vi "init.vi"(8 "error in (no error)":errorcluster, 10 "Variant":variant, 11 "Arduino Uno in":refnum<class "Arduino Uno.lvclass">) -> (0 "error out":errorcluster, 3 "Arduino Uno out":refnum<class "Arduino Uno.lvclass">)   [LabVIEW 2025, in "USB IO.lvlib" / "Arduino Uno.lvclass"]
uses:
  Arduino Uno.lvclass
  Arduino Uno.lvclass/Arduino Uno.ctl
  <vilib>/MakerHub/LINX/Public/Utilities/Open Serial.vi
  <vilib>/MakerHub/LINX/LMH-LINX.lvlib
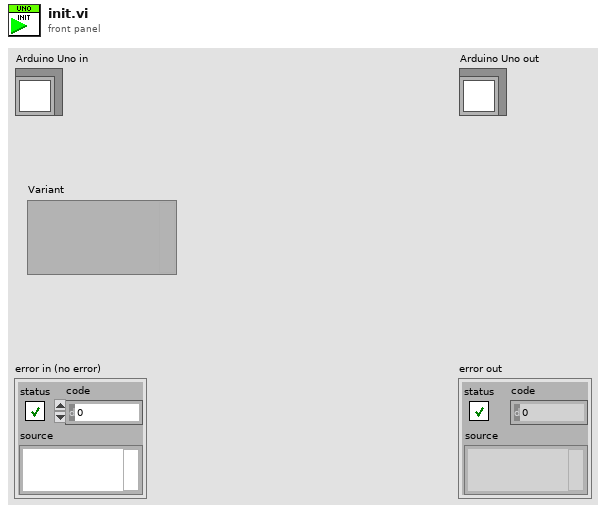
[diagram p1: front panel]
types:
  T1 = typedef "LMH-LINX.lvlib/LINX Ref.ctl" = cluster{"IO":T2, "Interface":T3, "LINX Device Config":T4}
  T2 = typedef "LMH-LINX.lvlib/Platform.ctl" = enum16{"Remote", "Local"}
  T3 = typedef "LMH-LINX.lvlib/Interface.ctl" = enum16{"Serial", "TCP"}
  T4 = typedef "LMH-LINX.lvlib/Device.lvlib/LINX Device Config.ctl" = cluster{"Interface":T3, "COM Port":refnum<visa-resource-name>, "TCP Configuration":T5, "Device Family":u8, "Device ID":u8, "Device Name":string, "TCP Ref":refnum<k5>, "Channels":T6}
  T5 = typedef "LMH-LINX.lvlib/Device.lvlib/TCP Config.ctl" = cluster{"IP Address":string, "Port":u16}
  T6 = typedef "LMH-LINX.lvlib/Channels.ctl" = cluster{"DI":u8[], "DO":u8[], "AI":u8[], "AO":u8[], "PWM":u8[], "QE":u8[], "UART":u8[], "I2C 2":u8[], "SPI":u8[], "CAN":u8[], "Servo":u8[], "AI Ref (V)":dbl, "AI Resolution (Bits)":u8, "AO Ref (V)":dbl, "AO Resolution (Bits)":u8}
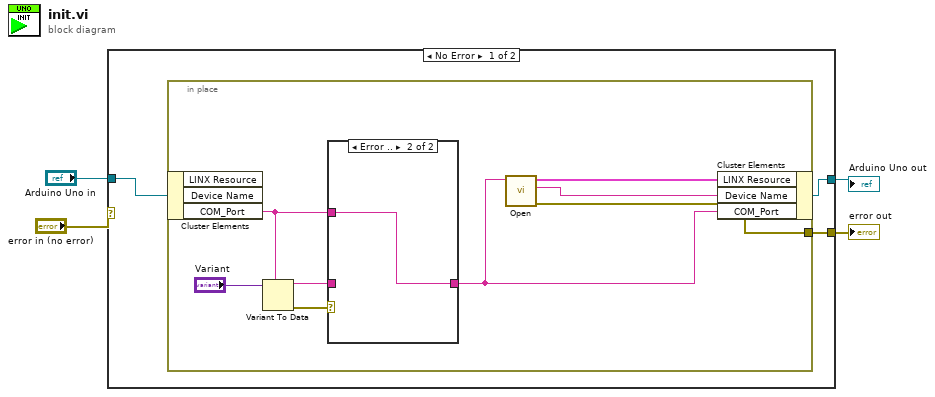
[diagram p0: block diagram]
diagram:
  n1 = case shown="No Error" "error in (no error)" {
    selector: "error in (no error)" -> [_ w18]
    tunnel: "Arduino Uno in" -> [w7 w19]
    tunnel: [w6 w18] -> w2
    tunnel: [w5 w19] -> w1
    frame No Error {
      n2 = in-place {
        in-place-border: [w14] -> w6
        n3 = in-place-cluster #1(w7) -> ("COM_Port"=w9:string)  [unwired: 2 out]
        n4 = Variant To Data(type=w9, Variant="Variant") -> (data=w10:string, error out=w11:errorcluster)  [unwired: 1 in]
        n5 = case shown="Error .." w11 {
          tunnel: w10 -> [w16 _]
          tunnel: [w16 w17] -> w8
          tunnel: w9 -> [_ w17]
          frame No Error {
          }
          frame Error {
          }
        }
        n6 = call-poly <vilib>:"Open.vi"("Serial Port"=w8) -> ("Error Out"=w14:errorcluster, "Device Name"=w13:string, "LINX Resource"=w15:T1)  [unwired: 8 in]
        n7 = in-place-cluster #1("LINX Resource"=w15, "Device Name"=w13, "COM_Port"=w8) -> (w5:refnum<class "Arduino Uno.lvclass">)
      }
    }
    frame Error {
    }
  }
  "error out" <- w2
  "Arduino Uno out" <- w1
